vi "TCP Write Read.vi"(8 "error in (no error)":errorcluster, 10 "Write Data":string, 11 "connection ID In":refnum<k5>) -> (0 "error out":errorcluster, 1 "Data Available?":bool, 2 "Read Data":string, 3 "connection ID Out":refnum<k5>)   [LabVIEW 2016, in "SLL Easy API via TCP.lvclass"]
doc: "This API does a sequential TCP Write and TCP Read. \n\nThis would be useful in places where we are sending a command to the TCP server and we want to wait and receive the data from the TCP Server."
uses:
  SLL Easy API via TCP.lvclass
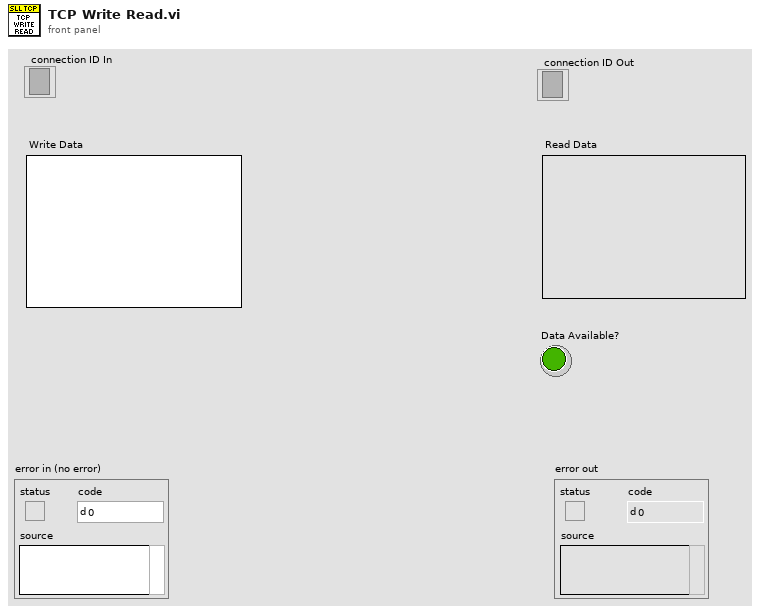
[diagram p1: front panel]
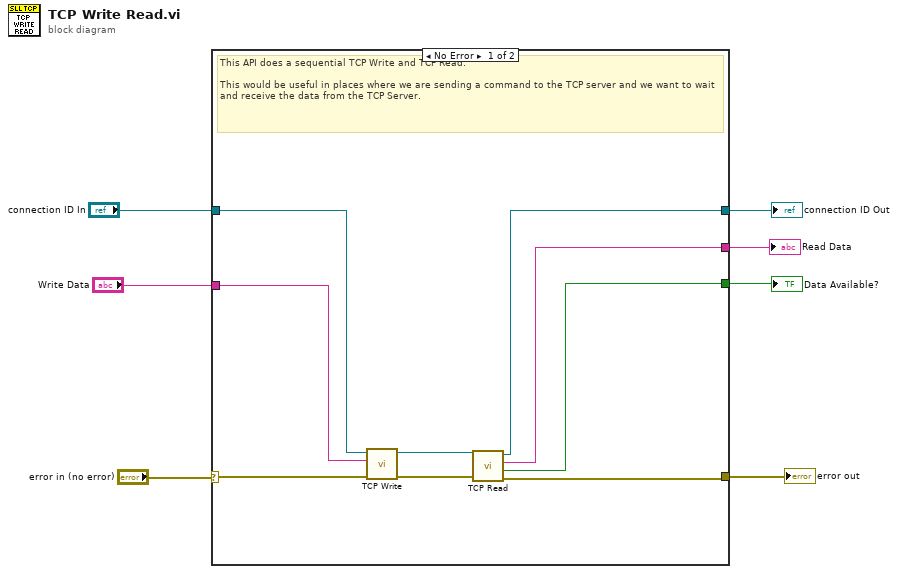
[diagram p0: block diagram]
diagram:
  n1 = case shown="No Error" "error in (no error)" {
    selector: "error in (no error)" -> [w16 w18]
    tunnel: "connection ID In" -> [w14 w17]
    tunnel: [w11 w18] -> w5
    tunnel: "Write Data" -> [w15 _]
    tunnel: [w9 w17] -> w3
    tunnel: [w10 _] -> w1
    tunnel: [w8 _] -> w2
    frame No Error {
      # "This API does a sequential TCP Write and TCP Read. \n\nThis would be useful in places where we are sending a command to the TCP server and we want to wait and receive the data from the TCP Server."
      n2 = call "TCP Write.vi"("error in (no error)"=w16, "Write Data"=w15, "connection ID In"=w14) -> ("error out"=w13:errorcluster, "connection ID Out"=w12:refnum<k5>)  [unwired: 7 in]
      n3 = call "TCP Read.vi"("error in (no error)"=w13, "Connection ID In"=w12) -> ("error out"=w11:errorcluster, "Data Available?"=w10:bool, "Read Data"=w8:string, "Connection ID Out"=w9:refnum<k5>)  [unwired: 6 in]
    }
    frame Error {
    }
  }
  "error out" <- w5
  "connection ID Out" <- w3
  "Read Data" <- w2
  "Data Available?" <- w1
